vi "Close.vi"(8 "error in (no error)":errorcluster, 10 "Msg in":T1, 11 "FakeCamera in":refnum<class "MoveDataFile.lvclass">) -> (0 "error out":errorcluster, 1 "new command":string, 2 "Msg out":T1, 3 "FakeCamera out":refnum<class "MoveDataFile.lvclass">)   [LabVIEW 2011, in "MoveDataFile.lvclass"]
uses:
  MoveDataFile.lvclass
  BaseDriver/BaseDriver.lvclass
  <vilib>/vision/driver/NI_Vision_Acquisition_Software.lvlib
  BaseDriver/DriverMsg.ctl
panel:
  out "error out 2":errorcluster
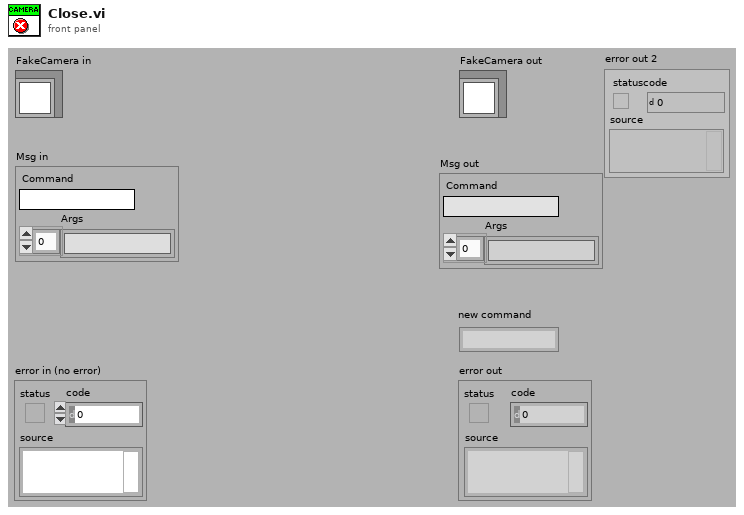
[diagram p1: front panel]
types:
  T1 = typedef "DriverMsg.ctl" = cluster{"Command":string, "Args":string[]}
  T2 = typedef "IMAQdx.ctl" = refnum<k21>
  T3 = typedef "IMAQ Image.ctl" = refnum<image>
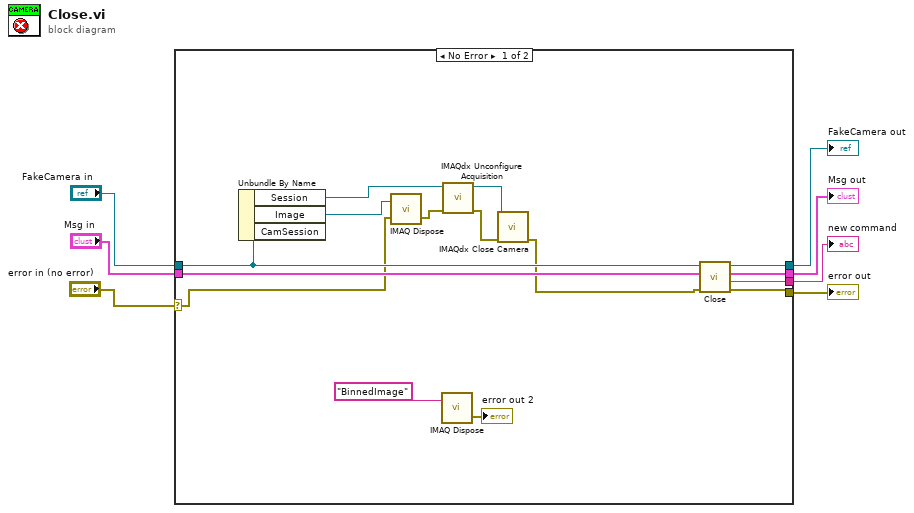
[diagram p0: block diagram]
diagram:
  n1 = case shown="No Error" "error in (no error)" {
    selector: "error in (no error)" -> [w15 w25]
    tunnel: [w22 w25] -> w7
    tunnel: [w21 _] -> w6
    tunnel: [w20 w24] -> w5
    tunnel: [w19 w23] -> w4
    tunnel: "Msg in" -> [w18 w24]
    tunnel: "FakeCamera in" -> [w17 w23]
    frame No Error {
      n2 = Unbundle By Name(w17) -> ("Session"=w12:T2, "Image"=w16:T3)  [unwired: 1 out]
      n3 = call "IMAQ Dispose"("Image"=w16, "error in (no error)"=w15) -> ("error out"=w11:errorcluster)  [unwired: 4 in]
      n4 = call "IMAQ Dispose"("Image"="BinnedImage" ("command or variable name")) -> ("error out"=→"error out 2":errorcluster)  [unwired: 5 in]
      n5 = call <vilib>:"IMAQdx Unconfigure Acquisition.vi"("error in"=w11, "Session In"=w12) -> ("error out"=w9:errorcluster, "Session Out"=w10:T2)  [unwired: 8 in]
      n6 = call <vilib>:"IMAQdx Close Camera.vi"("error in"=w9, "Session In"=w10) -> ("error out"=w8:errorcluster)  [unwired: 9 in]
      n7 = call-parent "Close.vi"("error in (no error)"=w8, "Msg in"=w18, "BaseDriver in"=w17) -> ("error out"=w22:errorcluster, "new command"=w21:string, "Msg out"=w20:T1, "BaseDriver out"=w19:refnum<class "MoveDataFile.lvclass">)  [unwired: 5 in]
    }
    frame Error {
    }
  }
  "error out" <- w7
  "FakeCamera out" <- w4
  "new command" <- w6
  "Msg out" <- w5
